vi "Initialize.vi"(11 "Swirly Vortex of Terror In":refnum<class "Swirly Vortex of Terror.lvclass">) -> (3 "Swirly Vortex of Terror Out":refnum<class "Swirly Vortex of Terror.lvclass">)   [LabVIEW 2015, in "Swirly Vortex of Terror.lvclass"]
uses:
  Swirly Vortex of Terror.lvclass
  Type Defs/Direction Enum.ctl
  Type.ctl
  Swirly Vortex of Terror.lvclass/Swirly Vortex of Terror.ctl
  Type Defs/SB Type Defs.lvlib
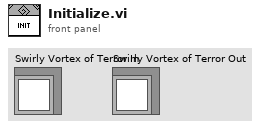
[diagram p1: front panel]
types:
  T1 = typedef "Swirly Vortex of Terror.lvclass/Type.ctl" = enum16{"Diagonal Starter", "Row Starter", "Vortex Eye", "Disciple", "Path Keeper", "Explorer"}
  T2 = typedef "SB Type Defs.lvlib/Direction Enum.ctl" = enum16{"NW", "N", "NE", "E", "SE", "S", "SW", "W"}
  T3 = typedef "Common.lvlib/Position.ctl" = cluster{"Column":i32, "Row":i32}
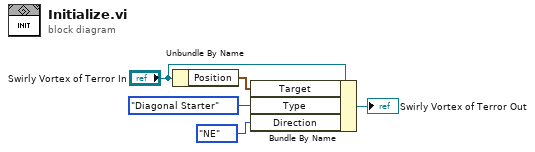
[diagram p0: block diagram]
diagram:
  n1 = Unbundle By Name("Swirly Vortex of Terror In") -> ("Position"=w1:T3)
  n2 = Bundle By Name(cluster="Swirly Vortex of Terror In", "Target"=w1, "Type"=Type."Diagonal Starter" ("Player. Type"), "Direction"=Direction_Enum."NE" ("Player.Direction")) -> (→"Swirly Vortex of Terror Out":refnum<class "Swirly Vortex of Terror.lvclass">)
